vi "Comm String Send Command.vi"(0 "niDTS Comm Serial in":refnum<class "niDTS Comm Serial.lvclass">, 5 "Command":string, 7 "Args":string, 11 "error in (no error)":errorcluster) -> (4 "niDTS Comm Serial out":refnum<class "niDTS Comm Serial.lvclass">, 6 "Response":string, 15 "error out":errorcluster)   [LabVIEW 2015, in "niDTS CommLib.lvlib" / "niDTS Comm Serial.lvclass"]
uses:
  niDTS Comm Serial.lvclass
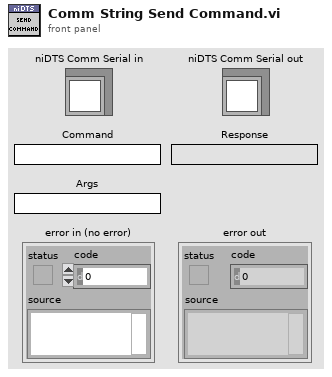
[diagram p1: front panel]
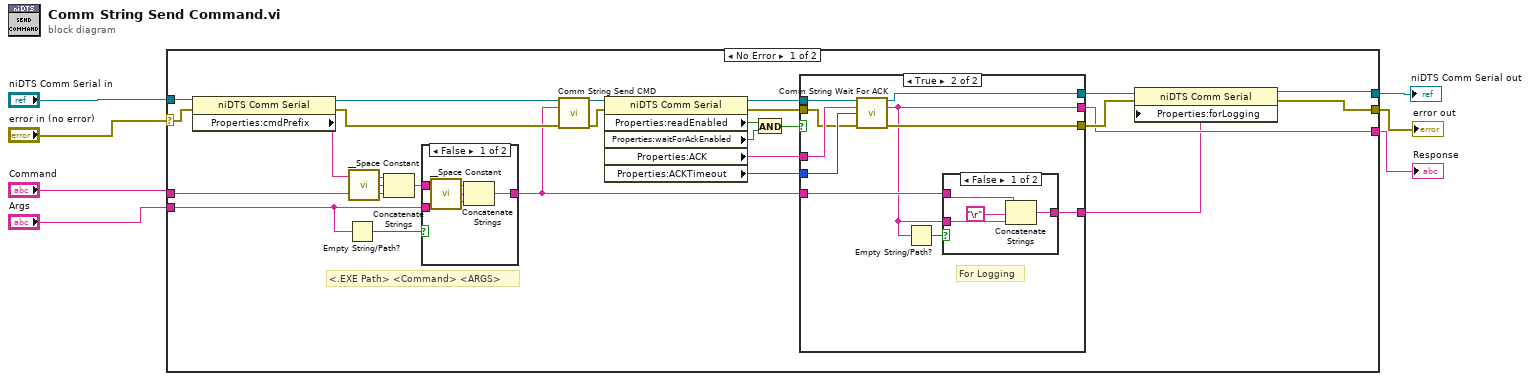
[diagram p0: block diagram]
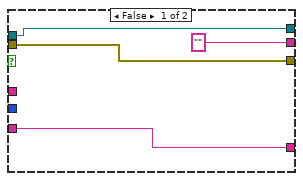
[diagram p2: hidden frame]
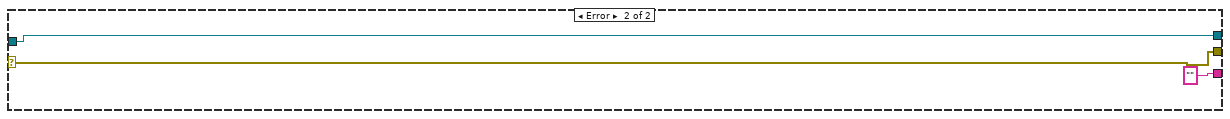
[diagram p5: hidden frame]
diagram:
  n1 = case shown="No Error" "error in (no error)" {
    selector: "error in (no error)" -> [w32 w58]
    tunnel: "niDTS Comm Serial in" -> [w33 w59]
    tunnel: "Command" -> [w27 _]
    tunnel: "Args" -> [w26 _]
    tunnel: [w10 "" ("Response")] -> w1
    tunnel: [w11 w59] -> w3
    tunnel: [w8 w58] -> w2
    frame No Error {
      # "<.EXE Path> <Command> <ARGS>"
      n2 = property class="niDTS Comm Serial"(reference=w33, error in=w32) -> (reference out=w25:refnum<class "niDTS Comm Serial.lvclass">, error out=w24:errorcluster, "Properties:cmdPrefix"=w28:string)
      n3 = Empty String/Path?(string/path=w26) -> (empty?=w29:bool)
      n4 = call "__Space Constant.vi"() -> ("String"=w31:string)
      n5 = Concatenate Strings(w28, w31, w27) -> (w30:string)
      n6 = case shown="False" w29 {
        tunnel: w30 -> [w56 w57]
        tunnel: [w53 w57] -> w14
        tunnel: w26 -> [w54 _]
        frame False {
          n7 = call "__Space Constant.vi"() -> ("String"=w55:string)
          n8 = Concatenate Strings(w56, w55, w54) -> (w53:string)
        }
        frame True {
        }
      }
      n9 = call-dynamic "Comm String Send CMD.vi"("niDTS Comm Serial in"=w25, "Command"=w14, "error in (no error)"=w24) -> ("niDTS Comm Serial out"=w23:refnum<class "niDTS Comm Serial.lvclass">, "error out"=w20:errorcluster)  [unwired: 11 in]
      n10 = property class="niDTS Comm Serial"(reference=w23, error in=w20) -> (reference out=w18:refnum<class "niDTS Comm Serial.lvclass">, error out=w17:errorcluster, "Properties:readEnabled"=w22:bool, "Properties:waitForAckEnabled"=w21:bool, "Properties:ACK"=w16:string, "Properties:ACKTimeout"=w15:i32)
      n11 = And(x=w22, y=w21) -> (x .and. y?=w19:bool)
      n12 = case shown="True" w19 {
        tunnel: w18 -> [w36 w47]
        tunnel: w17 -> [w35 w44]
        tunnel: w16 -> [_ w46]
        tunnel: w15 -> [_ w45]
        tunnel: ["" ("Response") w39] -> w10
        tunnel: [w36 w43] -> w13
        tunnel: [w35 w42] -> w12
        tunnel: w14 -> [w34 w40]
        tunnel: [w34 w38] -> w9
        frame False {
        }
        frame True {
          # "For Logging"
          n13 = call-dynamic "Comm String Wait For ACK.vi"("niDTS Comm Serial in"=w47, "ACK"=w46, "Timeout (ms)"=w45, "error in (no error)"=w44) -> ("niDTS Comm Serial out"=w43:refnum<class "niDTS Comm Serial.lvclass">, "Response"=w39:string, "error out"=w42:errorcluster)  [unwired: 8 in, 1 out]
          n14 = Empty String/Path?(string/path=w39) -> (empty?=w41:bool)
          n15 = case shown="False" w41 {
            tunnel: [w50 w52] -> w38
            tunnel: w40 -> [w49 w52]
            tunnel: w39 -> [w48 _]
            frame False {
              n16 = Concatenate Strings(w49, "\r", w48) -> (w50:string)
            }
            frame True {
            }
          }
        }
      }
      n17 = property class="niDTS Comm Serial"(reference=w13, error in=w12, "Properties:forLogging"=w9) -> (reference out=w11:refnum<class "niDTS Comm Serial.lvclass">, error out=w8:errorcluster)
    }
    frame Error {
    }
  }
  "error out" <- w2
  "niDTS Comm Serial out" <- w3
  "Response" <- w1
